vi "File_Insure Folder.vi"(0 "Folder":path) -> (2 "created path":path, 3 "Success":bool)   [LabVIEW 2020]
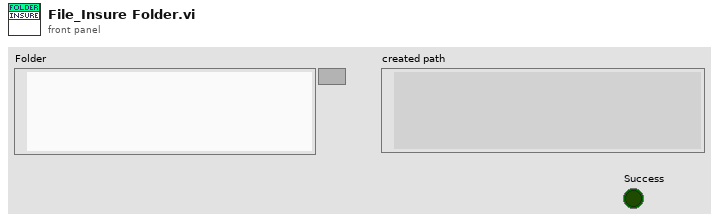
[diagram p1: front panel]
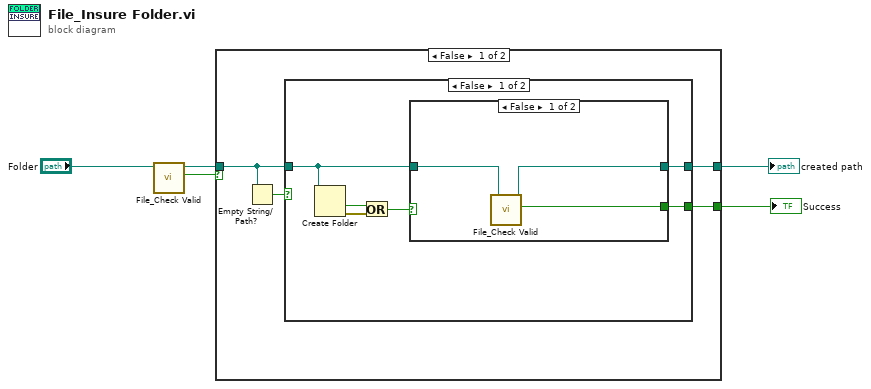
[diagram p0: block diagram]
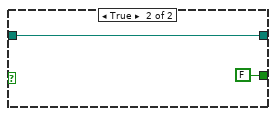
[diagram p2: hidden frame]
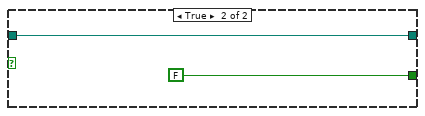
[diagram p3: hidden frame]
diagram:
  n1 = call "File_Check Valid.vi"("path"="Folder") -> ("dup path"=w4:path, "valid"=w5:bool)  [unwired: 4 in, 1 out]
  n2 = case shown="False" w5 {
    selector: w5 -> [_ w24]
    tunnel: w4 -> [w7 w23]
    tunnel: [w8 w24] -> w1
    tunnel: [w9 w23] -> w2
    frame False {
      n3 = Empty String/Path?(string/path=w7) -> (empty?=w6:bool)
      n4 = case shown="False" w6 {
        tunnel: [w15 w22] -> w9
        tunnel: [w14 FALSE ("file or folder exists?")] -> w8
        tunnel: w7 -> [w10 w22]
        frame False {
          n5 = Create Folder(path (use dialog)=w10) -> (cancelled=w11:bool, error out=w13:errorcluster)  [unwired: 2 in, 1 out]
          n6 = Or(x=w11, y=w13) -> (x .or. y?=w12:bool)
          n7 = case shown="False" w12 {
            tunnel: w10 -> [w18 w19]
            tunnel: [w16 w19] -> w15
            tunnel: [w17 FALSE ("file or folder exists?")] -> w14
            frame False {
              n8 = call "File_Check Valid.vi"("path"=w18) -> ("dup path"=w16:path, "valid"=w17:bool)  [unwired: 4 in, 1 out]
            }
            frame True {
            }
          }
        }
        frame True {
        }
      }
    }
    frame True {
    }
  }
  "created path" <- w2
  "Success" <- w1
